vi "Flow Array Convert.vi"(0 "Voltage":dynamicdata(waveform), 9 "Array - Numeric":dbl[](array[numeric]), 11 "error in (no error)":errorcluster) -> (4 "Result":dynamicdata(waveform), 15 "error out":errorcluster)   [LabVIEW 2015, in "SubVIs.lvlib"]
uses:
  SubVIs.lvlib
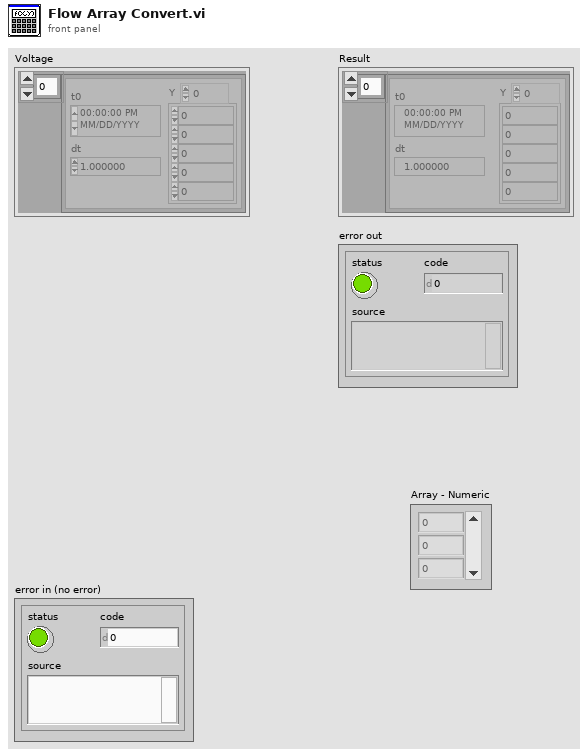
[diagram p1: front panel]
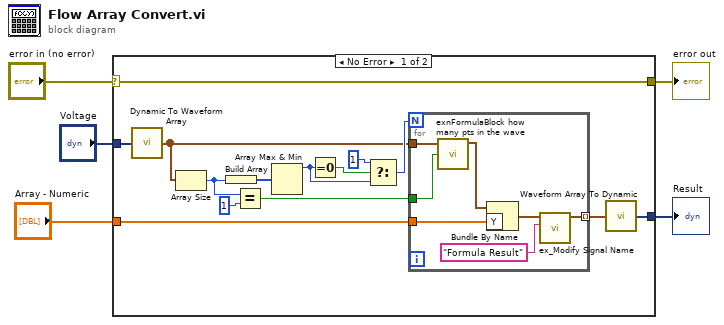
[diagram p0: block diagram]
diagram:
  n1 = case shown="No Error" "error in (no error)" {
    selector: "error in (no error)" -> [w7 w27]
    tunnel: [w8 _] -> w3
    tunnel: [w7 w27] -> w2
    tunnel: "Voltage" -> [w9 _]
    tunnel: "Array - Numeric" -> [w6 _]
    frame No Error {
      n2 = call <vilib>:"Dynamic To Waveform Array.vi"("Input"=w9) -> ("Output"=w10:waveform(dbl)[])  [unwired: 4 in]
      n3 = Array Size(array=w10) -> (size(s)=w17:i32)
      n4 = Build Array(w17) -> (w16:i32[])
      n5 = Equal?(x=w17, y=u8 1) -> (x = y?=w15:bool)
      n6 = Array Max & Min(array=w16) -> (max value=w13:i32)  [unwired: 3 out]
      n7 = Equal To 0?(x=w13) -> (x = 0?=w14:bool)
      n8 = Select(t=1, s=w14, f=w13) -> (s? t:f=w11:i32)
      n9 = for {
        N: w11 -> [_]
        tunnel: [w22] -> w19 mode=indexing
        tunnel: w15 -> [w25]
        tunnel: w10 -> [w24]
        tunnel: w6 -> [w20]
        n10 = call <vilib>:"exnFormulaBlock how many pts in the wave.vi"("Array"=w24, "Boolean"=w25) -> ("Waveform"=w26:waveform(dbl))  [unwired: 1 in, 3 out]
        n11 = Bundle By Name(cluster=w26, "Y"=w20) -> (w23:waveform(dbl))
        n12 = call <vilib>:"ex_Modify Signal Name.vi"("Name Modifier"="Formula Result", "waveform in"=w23) -> ("waveform out"=w22:waveform(dbl))  [unwired: 8 in, 1 out]
      }
      n13 = call <vilib>:"Waveform Array To Dynamic.vi"("Input"=w19) -> ("Output"=w8:dynamicdata)  [unwired: 4 in]
    }
    frame Error {
    }
  }
  "Result" <- w3
  "error out" <- w2
